vi "generateRampedSquareWave_fromAOparameters.vi"(0 "AO params":T1) -> (1 "Waveform":waveform(dbl), 2 "wflength":i32)   [LabVIEW 2015]
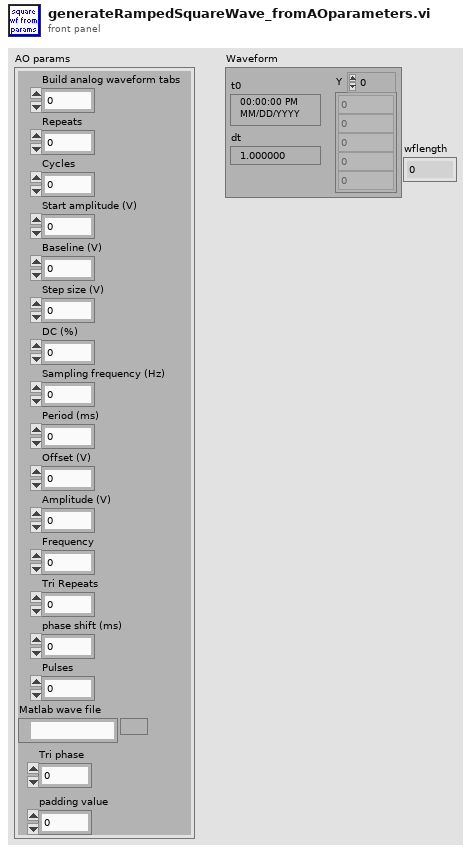
[diagram p1: front panel]
types:
  T1 = cluster{"Build analog waveform tabs":dbl, "Repeats":dbl, "Cycles":dbl, "Start amplitude (V)":dbl, "Baseline (V)":dbl, "Step size (V)":dbl, "DC (%)":dbl, "Sampling frequency (Hz)":dbl, "Period (ms)":dbl, "Offset (V)":dbl, "Amplitude (V)":dbl, "Frequency":dbl, "Tri Repeats":dbl, "phase shift (ms)":dbl, "Pulses":dbl, "Matlab wave file":path, "Tri phase":dbl, "padding value":dbl}
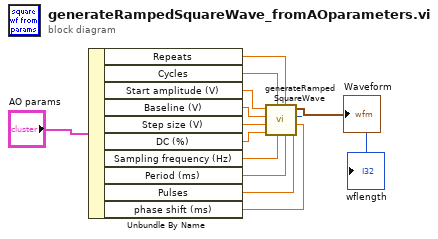
[diagram p0: block diagram]
diagram:
  n1 = Unbundle By Name("AO params") -> ("Repeats"=w6:dbl, "Cycles"=w7:dbl, "Start amplitude (V)"=w8:dbl, "Baseline (V)"=w9:dbl, "Step size (V)"=w10:dbl, "DC (%)"=w11:dbl, "Sampling frequency (Hz)"=w12:dbl, "Period (ms)"=w13:dbl, "Pulses"=w2:dbl, "phase shift (ms)"=w1:dbl)
  n2 = call "generateRampedSquareWave.vi"("pulses"=w2, "phase shift(ms)"=w1, "Period (ms)"=w13, "Repeats"=w6, "Sampling frequency (Hz)"=w12, "Cycles"=w7, "DC (%)"=w11, "Step size (V)"=w10, "Baseline (V)"=w9, "Start amplitude (V)"=w8) -> ("wflength"=→"wflength":i32, "Waveform"=→"Waveform":waveform(dbl))
